vi "Set RIO.vi"(8 "error in (no error)":errorcluster, 10 "ROI":T1, 11 "Camera Controller in":refnum<class "Camera Controller.lvclass">) -> (0 "error out":errorcluster, 3 "Camera Controller out":refnum<class "Camera Controller.lvclass">)   [LabVIEW 2022 SP3, in "Camera Controller.lvclass"]
uses:
  Camera Controller.lvclass
  Camera Controller.lvclass/Camera Controller.ctl
  Camera Data/Camera Data.lvclass
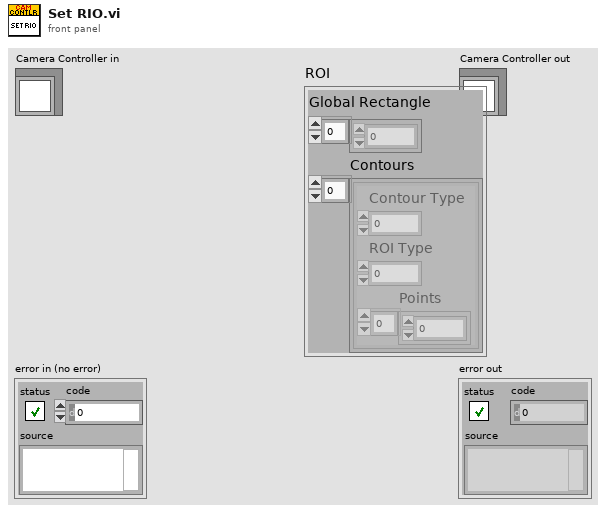
[diagram p1: front panel]
types:
  T1 = cluster{"Global Rectangle":i32[], "Contours":cluster{"Contour Type":u32, "ROI Type":u32, "Points":i32[]}[]}
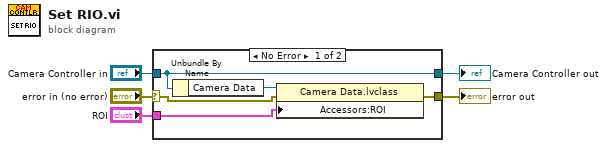
[diagram p0: block diagram]
diagram:
  n1 = case shown="No Error" "error in (no error)" {
    selector: "error in (no error)" -> [w7 w12]
    tunnel: [w6 w12] -> w4
    tunnel: [w8 w11] -> w2
    tunnel: "Camera Controller in" -> [w8 w11]
    tunnel: "ROI" -> [w9 _]
    frame No Error {
      n2 = Unbundle By Name(w8) -> ("Camera Data"=w10:refnum<data-value>)
      n3 = property class="Camera Data.lvclass"(reference=w10, error in=w7, "Accessors:ROI"=w9) -> (error out=w6:errorcluster)  [unwired: 1 out]
    }
    frame Error {
    }
  }
  "error out" <- w4
  "Camera Controller out" <- w2
